vi "Gate Facade.vi"(0 "Data In":T5={"Active"=FALSE, "Delay (ms)"=0.0, "Width (ms)"=50.0, "Ramp (ms)"=5.0}, 2 "Display State In":T3, 3 "Container State":T4) -> (6 "Data Out":T5={"Active"=FALSE, "Delay (ms)"=0.0, "Width (ms)"=50.0, "Ramp (ms)"=5.0}, 7 "Display State Out":T3, 8 "Action":T2)   [LabVIEW 2020, in "Gate Control.xctl"]
uses:
  Gate Control.xctl
  Gate Data.ctl
  <vilib>/_xctls/Container State.ctl
  Gate State.ctl
  <vilib>/_xctls/Action.ctl
  <vilib>/_xctls/XControlSupport.lvlib
panel:
  in  "Gate":T1
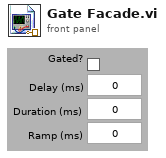
[diagram p1: front panel]
types:
  T1 = cluster{"Active":bool, "Delay (ms)":dbl, "Duration (ms)":dbl, "Ramp (ms)":dbl}
  T2 = typedef "XControlSupport.lvlib/Action.ctl" = cluster{"Data Changed?":bool, "State Changed?":bool, "Action Name":string}
  T3 = typedef "Gate Control.xctl/Gate State.ctl" = cluster{"Cluster":refnum<vi>}
  T4 = typedef "XControlSupport.lvlib/Container State.ctl" = cluster{"Indicator?":bool, "Run Mode?":bool, " Refnum":refnum<vi>}
  T5 = typedef "Gate Control.xctl/Gate Data.ctl" = cluster{"Active":bool, "Delay (ms)":dbl, "Width (ms)":dbl, "Ramp (ms)":dbl}
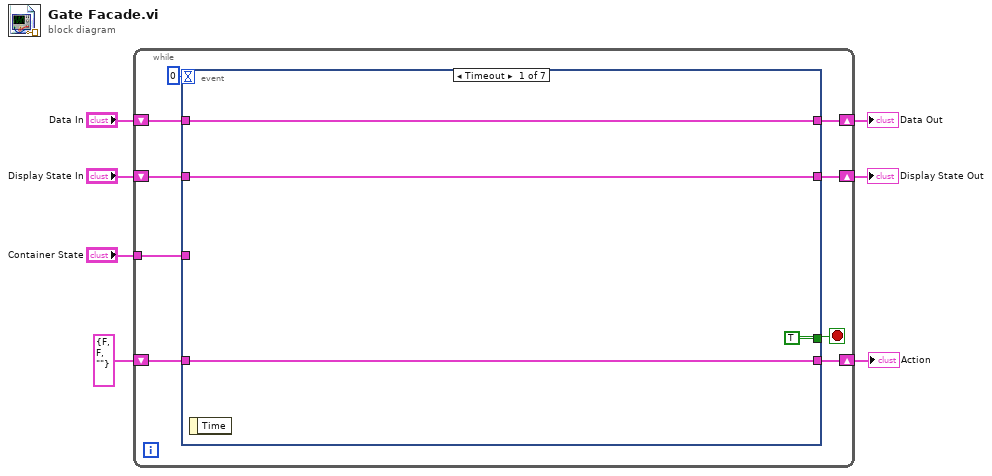
[diagram p0: block diagram]
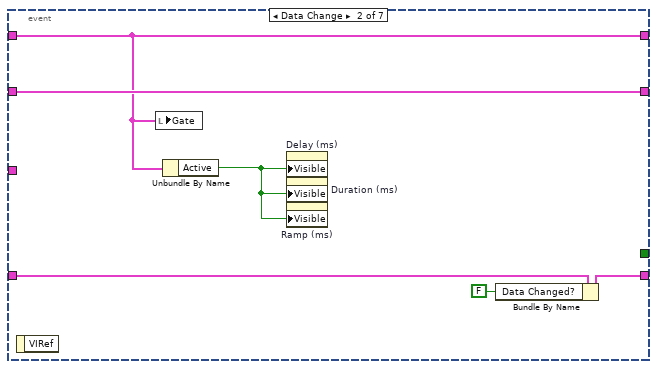
[diagram p2: hidden frame]
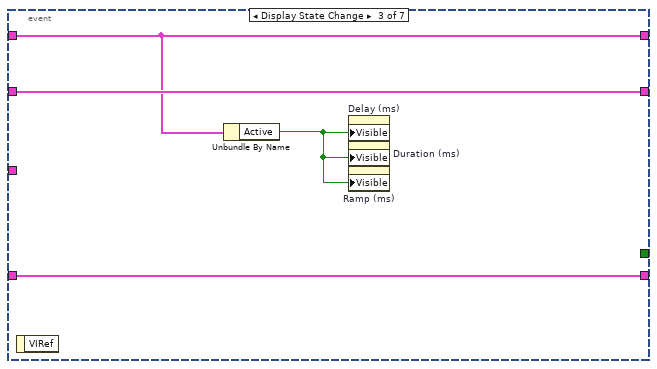
[diagram p3: hidden frame]
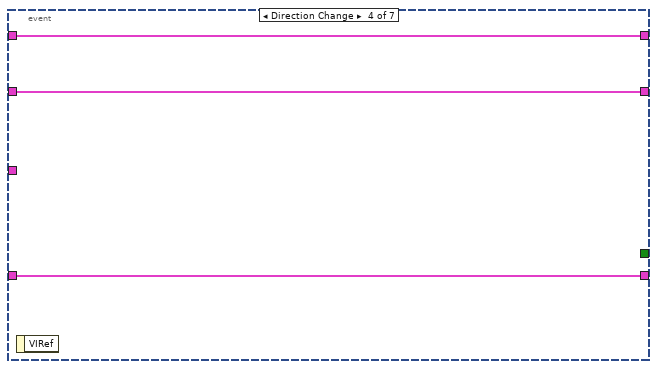
[diagram p4: hidden frame]
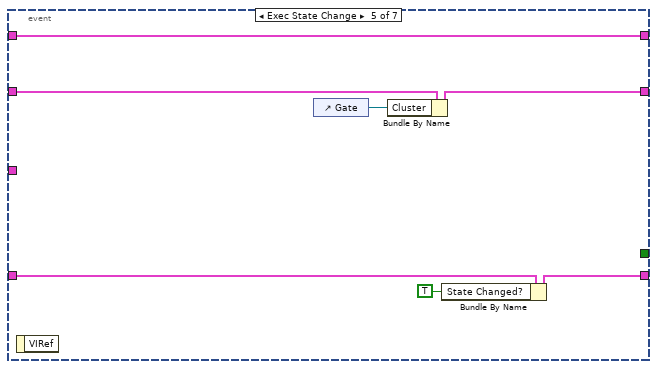
[diagram p5: hidden frame]
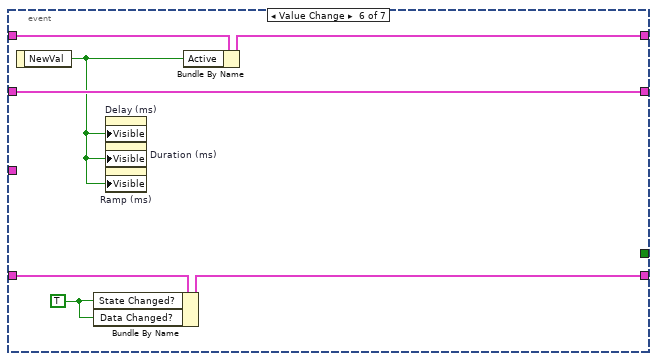
[diagram p6: hidden frame]
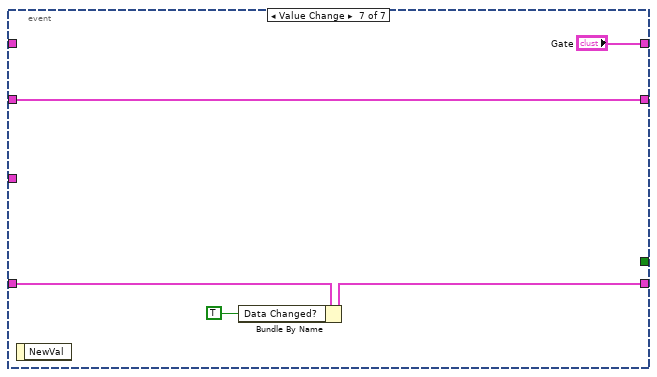
[diagram p7: hidden frame]
diagram:
  n1 = while {
    shift-right: [w15] -> w4
    shift-left: "Display State In" -> [w16]
    tunnel: "Container State" -> [w12]
    shift-right: [w10] -> w7
    shift-left: "Data In" -> [w11]
    shift-right: [w8] -> w2
    shift-left: T2 {"Data Changed?"=FALSE, "State Changed?"=FALSE, "Action Name"=""} ("Action") -> [w9]
    stop <- w14 stop-if-true
    n2 = event shown="[0] Timeout" {
      selector: _ -> [_ _ _ _ _ _ _]
      dyn-events: _ -> [_ _ _ _ _ _ _]
      timeout: 0 -> [_ _ _ _ _ _ _]
      tunnel: w16 -> [w18 w26 w30 w33 w40 w47 w51]
      tunnel: [w18 w26 w30 w33 w37 w47 w51] -> w15
      tunnel: [TRUE _ _ _ _ _ _] -> w14
      tunnel: w12 -> [_ _ _ _ _ _ _]
      tunnel: w11 -> [w17 w24 w27 w32 w39 w43 _]
      tunnel: [w17 w24 w27 w32 w39 w44 "Gate"] -> w10
      tunnel: [w19 w23 w29 w31 w35 w45 w49] -> w8
      tunnel: w9 -> [w19 w25 w29 w31 w38 w46 w50]
      event Timeout {
        n3 = event-data() -> ()  [unwired: 1 in, 1 out]
      }
      event Data Change {
        n4 = event-data() -> ()  [unwired: 1 in, 1 out]
        n5 = local write "Gate"(w24) -> ()
        n6 = Unbundle By Name(w24) -> ("Active"=w21:bool)
        n7 = property on="Delay (ms)" class="DigNum (strict)"("Visible"=w21) -> ()  [unwired: 2 in, 2 out]
        n8 = property on="Duration (ms)" class="DigNum (strict)"("Visible"=w21) -> ()  [unwired: 2 in, 2 out]
        n9 = property on="Ramp (ms)" class="DigNum (strict)"("Visible"=w21) -> ()  [unwired: 2 in, 2 out]
        n10 = Bundle By Name(cluster=w25, "Data Changed?"=FALSE) -> (w23:T2)
      }
      event Display State Change {
        n11 = event-data() -> ()  [unwired: 1 in, 1 out]
        n12 = Unbundle By Name(w27) -> ("Active"=w28:bool)
        n13 = property on="Delay (ms)" class="DigNum (strict)"("Visible"=w28) -> ()  [unwired: 2 in, 2 out]
        n14 = property on="Duration (ms)" class="DigNum (strict)"("Visible"=w28) -> ()  [unwired: 2 in, 2 out]
        n15 = property on="Ramp (ms)" class="DigNum (strict)"("Visible"=w28) -> ()  [unwired: 2 in, 2 out]
      }
      event Direction Change {
        n16 = event-data() -> ()  [unwired: 1 in, 1 out]
      }
      event Exec State Change {
        n17 = event-data() -> ()  [unwired: 1 in, 1 out]
        n18 = control-ref of="Gate"() -> (w36:refnum<vi>)
        n19 = Bundle By Name(cluster=w40, "Cluster"=w36) -> (w37:T3)
        n20 = Bundle By Name(cluster=w38, "State Changed?"=TRUE) -> (w35:T2)
      }
      event "Gate.Active": Value Change {
        w41 = TRUE ("State Changed?")
        n21 = event-data() -> ("NewVal"=w42:bool)  [unwired: 1 in]
        n22 = Bundle By Name(cluster=w46, "State Changed?"=w41, "Data Changed?"=w41) -> (w45:T2)
        n23 = property on="Delay (ms)" class="DigNum (strict)"("Visible"=w42) -> ()  [unwired: 2 in, 2 out]
        n24 = property on="Duration (ms)" class="DigNum (strict)"("Visible"=w42) -> ()  [unwired: 2 in, 2 out]
        n25 = property on="Ramp (ms)" class="DigNum (strict)"("Visible"=w42) -> ()  [unwired: 2 in, 2 out]
        n26 = Bundle By Name(cluster=w43, "Active"=w42) -> (w44:T5)
      }
      event "Gate.Delay (ms)", "Gate.Duration (ms)", "Gate.Ramp (ms)": Value Change {
        n27 = event-data() -> ()  [unwired: 1 in, 1 out]
        n28 = Bundle By Name(cluster=w50, "Data Changed?"=TRUE) -> (w49:T2)
      }
    }
  }
  "Display State Out" <- w4
  "Data Out" <- w7
  "Action" <- w2
